vi "Read motor_param.vi"(8 "error in (no error)":errorcluster, 11 "SMSD in":refnum<class "SMSD.lvclass">) -> (0 "error out":errorcluster, 2 "MOTOR_PARAM":T1={"DRIVER_MODE"=enum."VOLTAGE", "MOTOR_Type_42"=enum."Unknown", "MICROSTEPPING"=enum."1", "WORK_CURRENT"=enum."0.1A", "STOP_CURRENT"=enum."25%"}, 3 "SMSD out":refnum<class "SMSD.lvclass">)   [LabVIEW 2021, in "SMSD.lvclass"]
uses:
  SMSD.lvclass
  Ctl/MOTOR_PARAM.ctl
  Ctl/DRIVER_MODE.ctl
  Ctl/MOTOR_Type_42.ctl
  Ctl/MICROSTEPPING.ctl
  Ctl/WORK_CURRENT.ctl
  Ctl/STOP_CURRENT.ctl
  SMSD.lvclass/SMSD.ctl
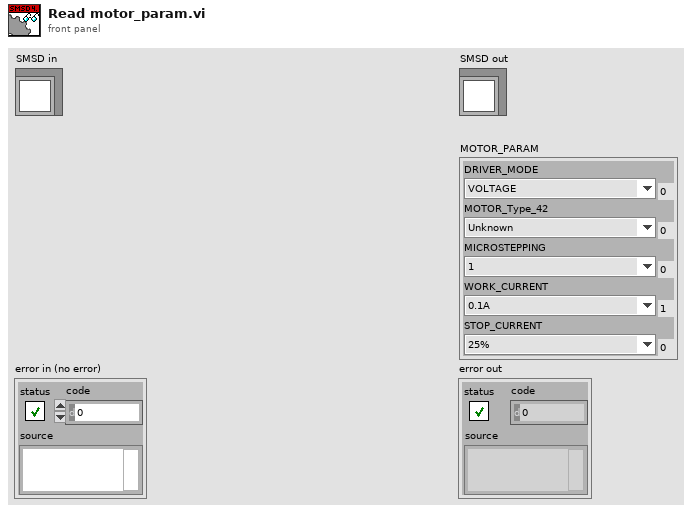
[diagram p1: front panel]
types:
  T1 = typedef "SMSD.lvclass/MOTOR_PARAM.ctl" = cluster{"DRIVER_MODE":T2, "MOTOR_Type_42":T3, "MICROSTEPPING":T4, "WORK_CURRENT":T5, "STOP_CURRENT":T6}
  T2 = typedef "SMSD.lvclass/DRIVER_MODE.ctl" = enum16{"VOLTAGE", "CURRENT"}
  T3 = typedef "SMSD.lvclass/MOTOR_Type_42.ctl" = enum16{"Unknown", "FL42STH33-1334 1.8 deg", "FL42STH33-1334 0.9 deg", "FL42STH38-1206 0.9 deg", "FL42STH38-1684 1.8 deg", "FL42STH38-1684 0.9 deg", "FL42STH47-1206 1.8 deg", "FL42STH47-1684 1.8 deg", "FL42STH47-1684 0.9 deg", "FL42STH60-1206 1.8 deg", "FL42STH60-1206 0.9 deg", "FL57ST41-1564 1.8 deg", "FL57ST76-1006 1.8 deg", "FL57ST76-1506 1.8 deg", "FL57STH41-1006 1.8 deg", "FL57STH41-1006 0.9 deg", "FL57STH41-2804 1.8 deg", "FL57STH41-2804 0.9 deg", "FL57STH51-1006 1.8 deg", "FL57STH51-2804 1.8 deg", "FL57STH51-2804 0.9 deg", "FL57STH56-1006 1.8 deg", "FL57STH56-2006 1.8 deg", "FL57STH56-2804 1.8 deg", "FL57STH76-1006 1.8 deg", "FL57STH76-2804 1.8 deg", "FL57STH76-2804 0.9 deg", "FL60STH65-2008 1.8 deg parallel", "FL60STH65-2008 1.8 deg serial", "FL60STH86-2008 1.8 deg parallel", "FL60STH86-2008 1.8 deg serial", "FL86STH65-2808 1.8 deg parallel", "FL86STH65-2808 1.8 deg serial", "FL86STH80-4208 1.8 deg parallel", "FL86STH80-4208 1.8 deg serial", "FL86STH118-4208 1.8 deg parallel", "FL86STH118-4208 1.8 deg serial", "FL86STH156-4208 1.8 deg parallel", "FL86STH156-4208 1.8 deg serial", "ДШ3934-0,3А", "ДШ2851-0,7А", "ДШ4248-1,7A", "ДШ5776-3,0А", "ДШ57112-3,0А", "ДШ8665-3,0А", "ДШ8682-4,5А"}
  T4 = typedef "SMSD.lvclass/MICROSTEPPING.ctl" = enum16{"1", "1/2", "1/4", "1/8", "1/16", "1/32", "1/64", "1/128"}
  T5 = typedef "SMSD.lvclass/WORK_CURRENT.ctl" = enum16{"0.0A", "0.1A", "0.2A", "0.3A", "0.4A", "0.5A", "0.6A", "0.7A", "0.8A", "0.9A", "1.0A", "1.1A", "1.2A", "1.3A", "1.4A", "1.5A", "1.6A", "1.7A", "1.8A", "1.9A", "2.0A", "2.1A", "2.2A", "2.3A", "2.4A", "2.5A", "2.6A", "2.7A", "2.8A", "2.9A", "3.0A", "3.1A", "3.2A", "3.3A", "3.4A", "3.5A", "3.6A", "3.7A", "3.8A", "3.9A", "4.0A", "4.1A", "4.2A"}
  T6 = typedef "SMSD.lvclass/STOP_CURRENT.ctl" = enum16{"25%", "50%", "75%", "100%"}
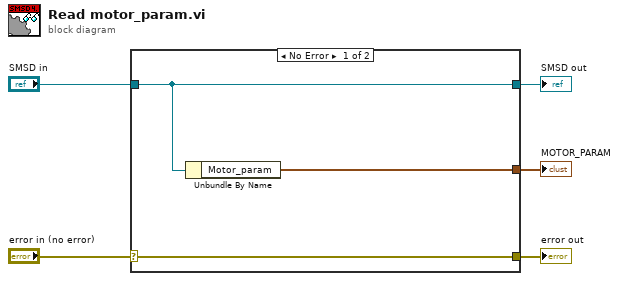
[diagram p0: block diagram]
diagram:
  n1 = case shown="No Error" "error in (no error)" {
    selector: "error in (no error)" -> [w8 w9]
    tunnel: [w8 w9] -> w4
    tunnel: [w7 w10] -> w2
    tunnel: "SMSD in" -> [w7 w10]
    tunnel: [w6 _] -> w1
    frame No Error {
      n2 = Unbundle By Name(w7) -> ("Motor_param"=w6:T1)
    }
    frame Error {
    }
  }
  "error out" <- w4
  "SMSD out" <- w2
  "MOTOR_PARAM" <- w1
